vi "closeMeas.vi"(8 "error in (no error)":errorcluster, 11 "FPGA VI (in) 2":T1) -> ()   [LabVIEW 2017]
uses:
  <vilib>/rvi/interface/nirviCloseFPGA/nirviCloseFPGA.xnode
  FPGA Bitfiles/PVemulator_FPGATarget2_IpDFT-only-DC2x9_aEit3VyAdvg.lvbitx
  <vilib>/FPGAPlugInAG/cRIO-9118/niLvFpga_Close_cRIO-9118.vi
  FPGA Bitfiles/FPGA.ctl
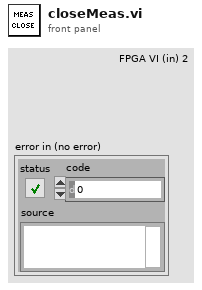
[diagram p1: front panel]
types:
  T1 = typedef "FPGA.ctl" = refnum<k20>
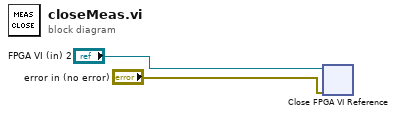
[diagram p0: block diagram]
diagram:
  n1 = xnode "Close FPGA VI Reference"("FPGA VI Reference In"="FPGA VI (in) 2", "error in"="error in (no error)") -> ()  [unwired: 1 out]
